vi "Main.vi"() -> ()   [LabVIEW 2026]
doc: "This template is for the Queued Message Handler design pattern.\n\nThe Event Handling Loop generates messages based on user interface actions.\n\nThe Message Handling Loop processes messages generated by the Event Handling Loop, or by other messages. The messages are string values, so new messages can be added easily to the Message Cases case structure in the Message Handling Loop. Each message cluster can also provide an optional value for Message Data, which is a variant that can be converted to whatever message-specific data is required."
uses:
  SubVIs/Controls/PCO_Config.ctl
  SubVIs/Controls/UI Data.ctl
  <instrlib>/PCO_SDK/File Group 0/vi.lib/Excelitas PCO GmbH/pco.labview/camera/Camera.lvclass
  <instrlib>/PCO_SDK/File Group 0/vi.lib/Excelitas PCO GmbH/pco.labview/camera/Controls/binning.ctl
  SubVIs/QMH/Message Queue/Enqueue Message (Single).vi
  SubVIs/QMH/Message Queue/Message Queue.lvlib
  SubVIs/QMH/User Event - Stop/User Event - Stop.lvlib
panel:
  out "Image 2":T1(plugin-control)
  in  "Stop live":bool
  out "rawImage":u16[][](array[numeric])
  out "Recording On":bool
  in  "FFT?":bool
  in  "Grab":bool
  in  "Live":bool
  in  "PCO_Config":T2={"Exposure time (s)"=0.1, "TriggerMode"=0, "ROI X0"=1, "ROI Y0"=1, "ROI X1"=2048, "ROI Y1"=2048, "Binning"=1} {"TriggerMode" items=["auto sequence", "software trigger", "external exposure start", "external exposure control"]}
  out "Image dimensions (px)":dbl[](array[numeric])=[2048.0, 2048.0]
  out "description":T3={"serial"=14401698, "type"=5632, "sub_type"=0, "interface_type"=8, "bit_resolution"=16, "min_exposure_time_s"=2.1e-05, "max_exposure_time_s"=5.0, "min_exposure_step_s"=1.2136e-05, "min_delay_time_s"=0.0, "max_delay_time_s"=5.0, "min_delay_step_s"=2.5e-08, "min_width"=64, "min_height"=16, "max_width"=2048, "max_height"=2048, "roi_step_horz"=32, "roi_step_vert"=8, "roi_symmetric_horz"=FALSE, "roi_symmetric_vert"=FALSE, "has_timestamp_mode"=TRUE, "has_timestamp_mode_ascii_only"=TRUE, "pixelrate_vec"=[44000000, 0, 0, 0], "has_acquire_mode"=TRUE, "has_ext_acquire_mode"=FALSE, "has_metadata_mode"=TRUE, "has_ram"=FALSE, "binning_horz_vec"=[1, 2, 4], "binning_vert_vec"=[1, 2, 4], "has_average_binning"=FALSE, "pixel_format_vec"=[1], "has_trigger_mode_extexpctrl"=TRUE} {"interface_type" items=["FireWire"=1, "GenICam"=3, "GigE"=5, "USB"=6, "CameraLinkME4"=7, "USB3"=8, "CLHS"=11, "All"=65535]}
  out "Current task":string="\"Exit\" button pressed"
  in  "Exit":bool
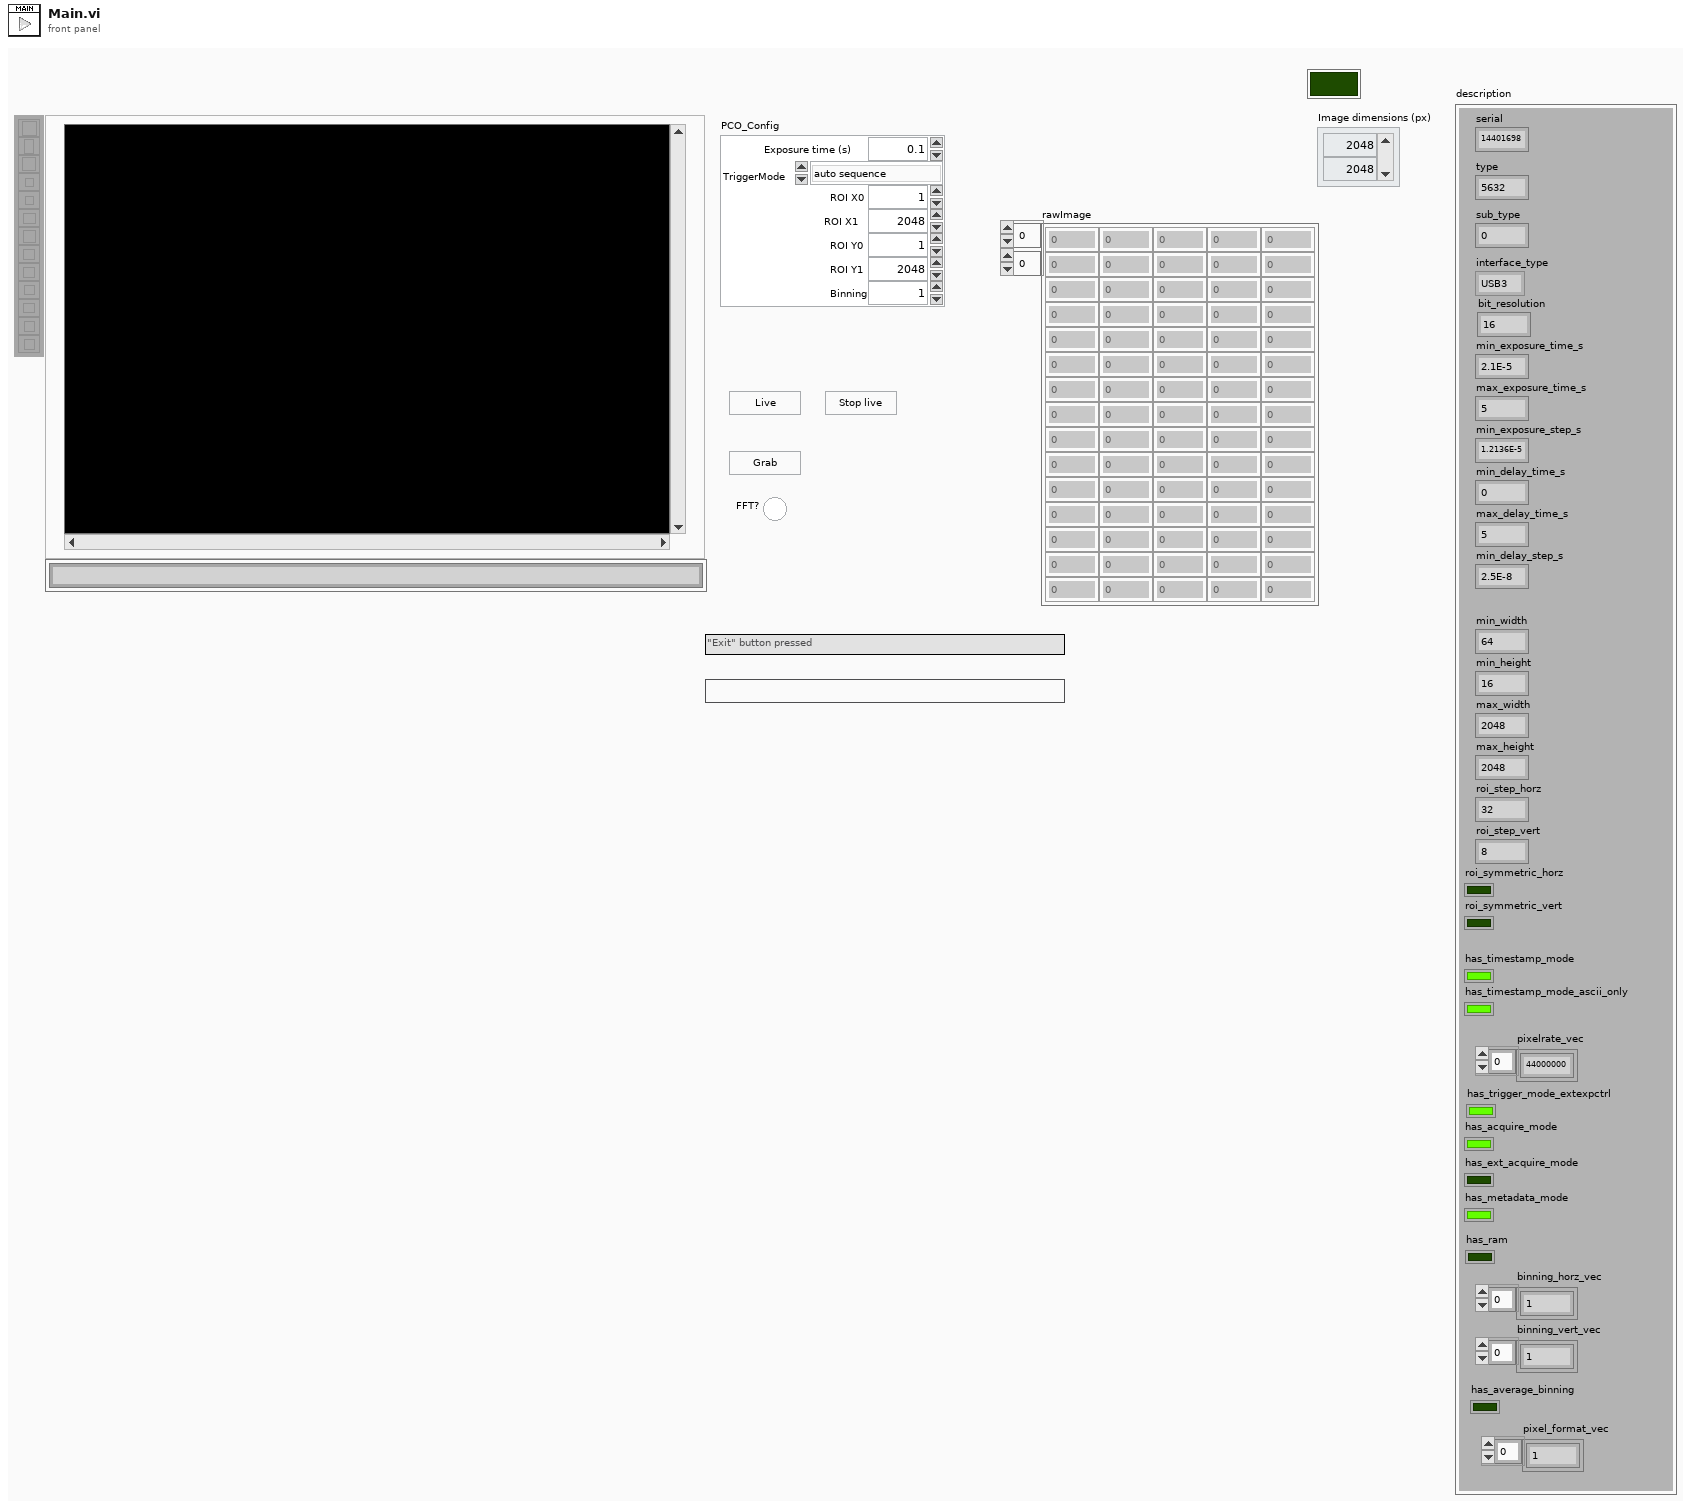
[diagram p1: front panel]
types:
  T1 = typedef "IMAQ Image.ctl" = refnum<image>
  T2 = typedef "PCO_Config.ctl" = cluster{"Exposure time (s)":dbl, "TriggerMode":u16, "ROI X0":u16, "ROI Y0":u16, "ROI X1":u16, "ROI Y1":u16, "Binning":u8}
  T3 = cluster{"serial":u32, "type":u16, "sub_type":u16, "interface_type":u16, "bit_resolution":u16, "min_exposure_time_s":dbl, "max_exposure_time_s":dbl, "min_exposure_step_s":dbl, "min_delay_time_s":dbl, "max_delay_time_s":dbl, "min_delay_step_s":dbl, "min_width":u64, "min_height":u64, "max_width":u64, "max_height":u64, "roi_step_horz":u64, "roi_step_vert":u64, "roi_symmetric_horz":bool, "roi_symmetric_vert":bool, "has_timestamp_mode":bool, "has_timestamp_mode_ascii_only":bool, "pixelrate_vec":u32[], "has_acquire_mode":bool, "has_ext_acquire_mode":bool, "has_metadata_mode":bool, "has_ram":bool, "binning_horz_vec":u16[], "binning_vert_vec":u16[], "has_average_binning":bool, "pixel_format_vec":u32[], "has_trigger_mode_extexpctrl":bool}
  T4 = typedef "UI Data.ctl" = cluster{"Data Display Ref":refnum<vi>, "Exit Button Ref":refnum<vi>, "Message":string}
  T5 = typedef "Message Queue.lvlib/All Message Queues.ctl" = cluster{"UI":refnum<queue>, "Camera loop":refnum<queue>, "Display loop":refnum<queue>}
  T6 = typedef "Camera.lvclass/binning.ctl" = cluster{"vert":u16, "horz":u16, "mode":u16}
  T7 = cluster{"exposure_time_s":dbl, "delay_time_s":dbl, "roi":cluster{"x0":u64, "y0":u64, "x1":u64, "y1":u64}, "timestamp_mode":u16, "pixelrate":u32, "trigger_mode":u16, "acquire_mode":u16, "metadata_mode":u16, "noisefilter_mode":u16, "pixel_format":u32, "binning":T6, "auto_exposure":cluster{"region":u16, "min_exposure_s":dbl, "max_exposure_s":dbl}}
  T8 = enum16{"sequence", "sequence non blocking", "ring buffer", "fifo", "sequence_dpcore", "sequence_non_blocking_dpcore", "ring_buffer_dpcore", "fifo_dpcore", "tif", "multitif", "pcoraw", "b16", "dicom", "multidicom", "camram_ring", "camram_segment"}
  T9 = enum16{"Undefined", "Mono8", "Mono16", "BGRA8", "RGBA8", "BGRA16", "RGBA16", "CompressedMono8"}
  T10 = typedef "Image Type" = u32
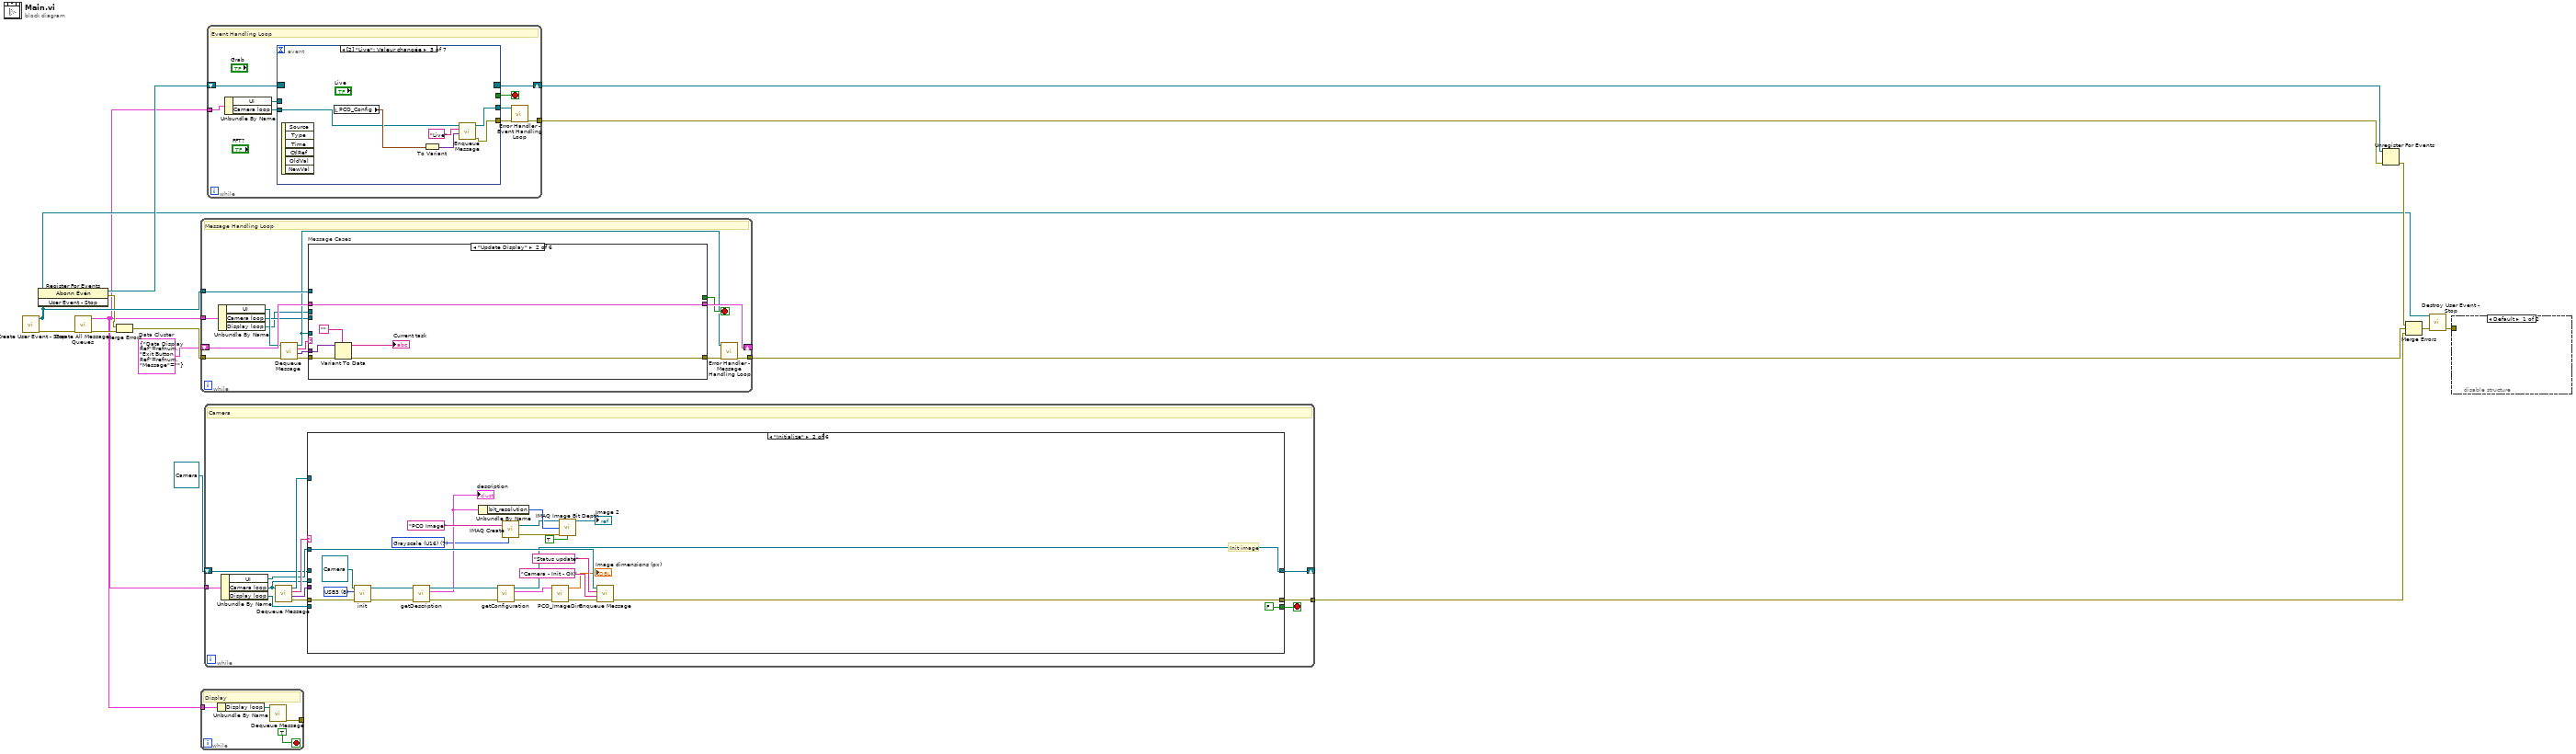
[diagram p0: block diagram]
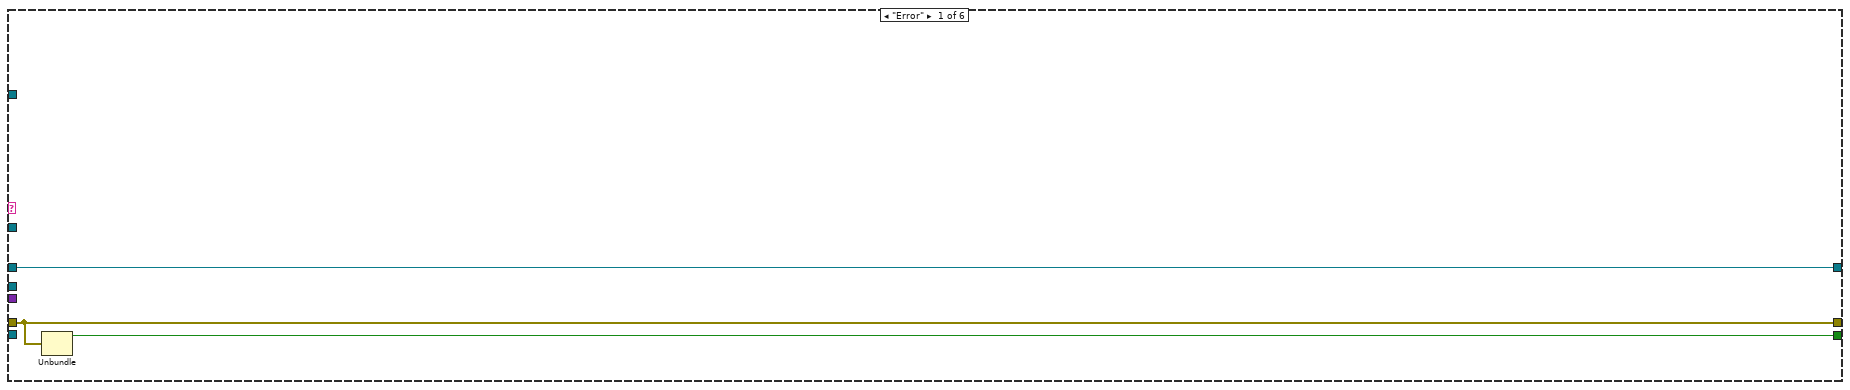
[diagram p2: hidden frame]
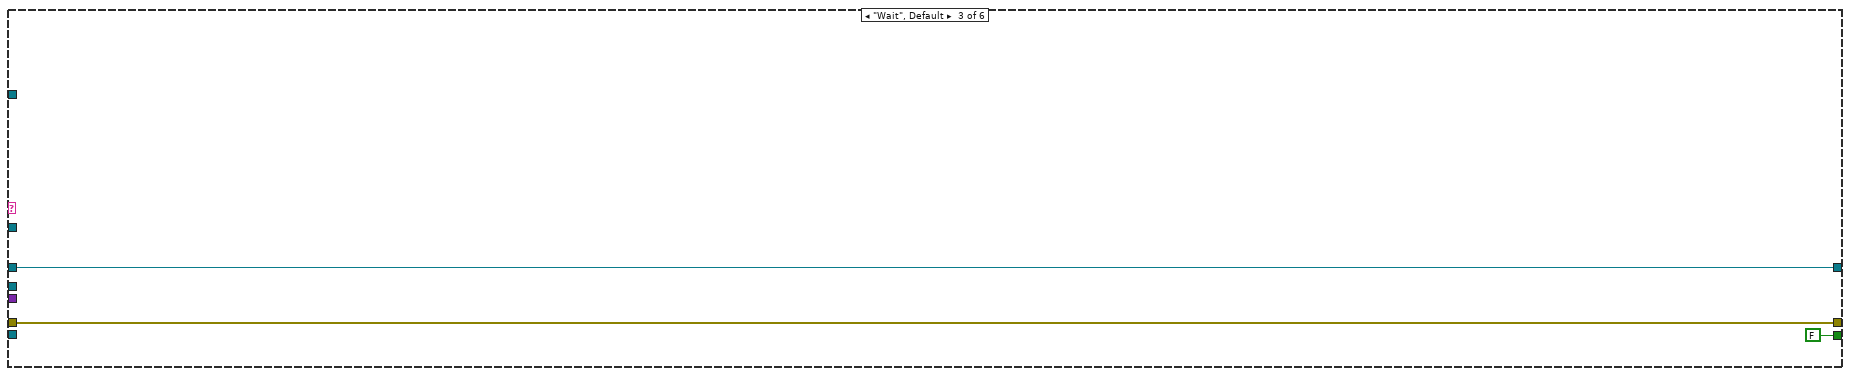
[diagram p3: hidden frame]
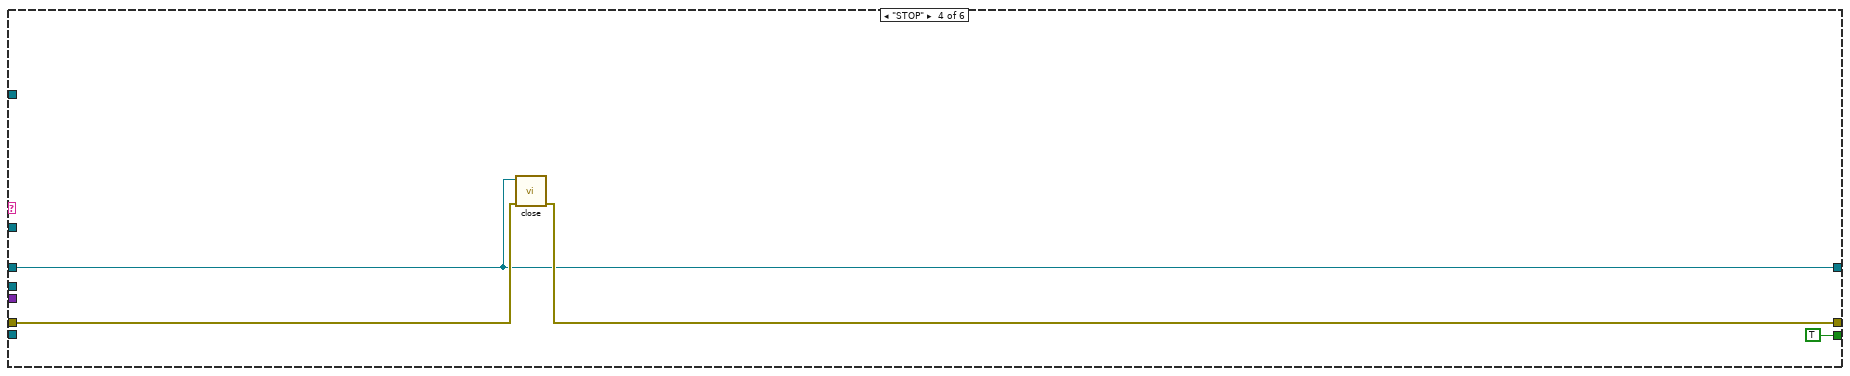
[diagram p4: hidden frame]
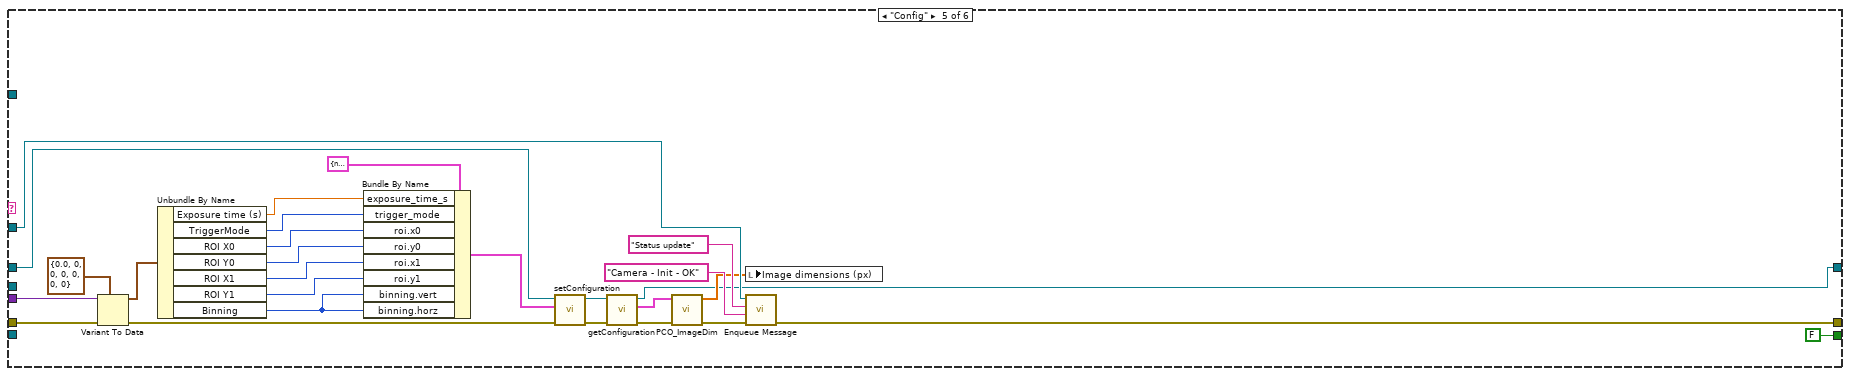
[diagram p5: hidden frame]
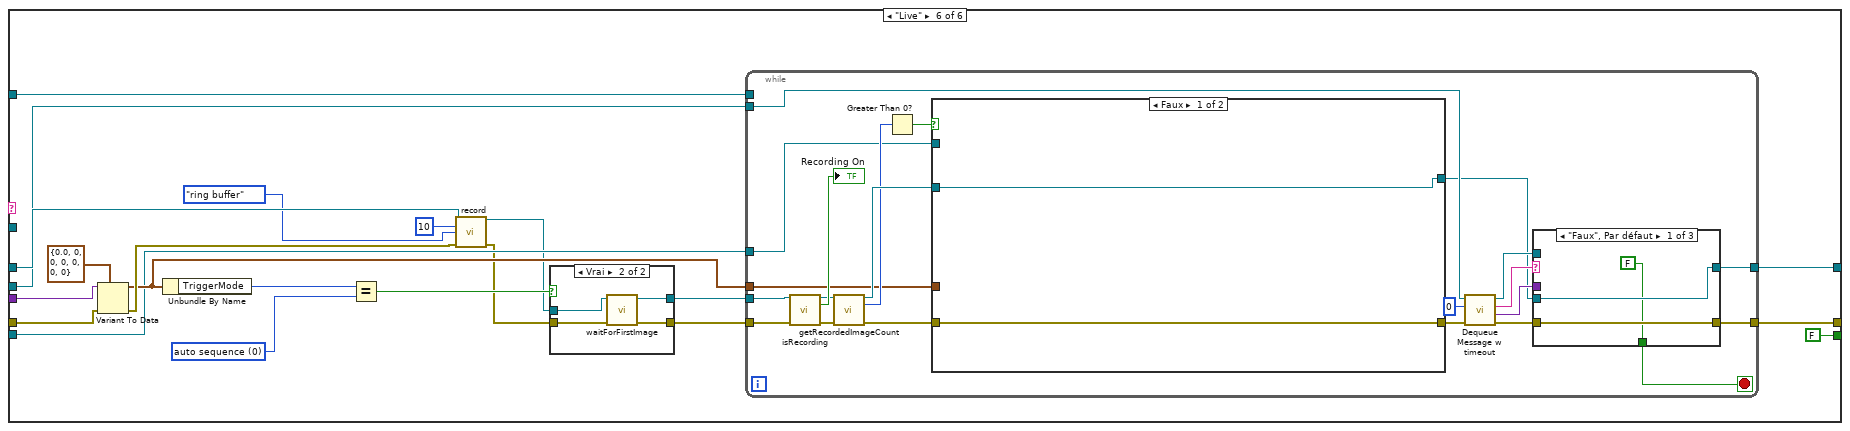
[diagram p6: hidden frame]
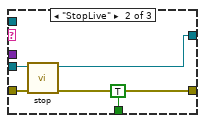
[diagram p7: hidden frame]
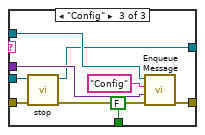
[diagram p8: hidden frame]
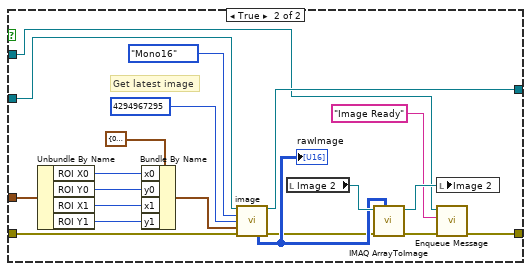
[diagram p9: hidden frame]
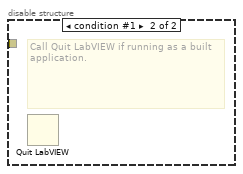
[diagram p11: hidden frame]
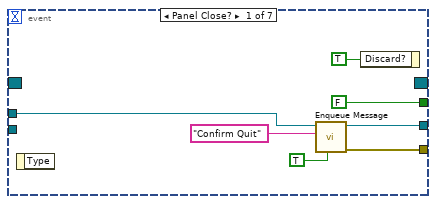
[diagram p12: hidden frame]
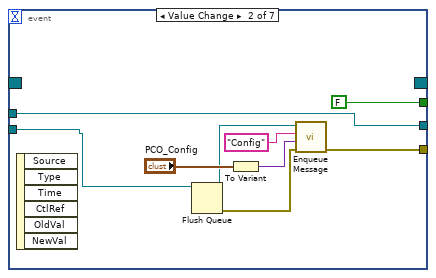
[diagram p13: hidden frame]
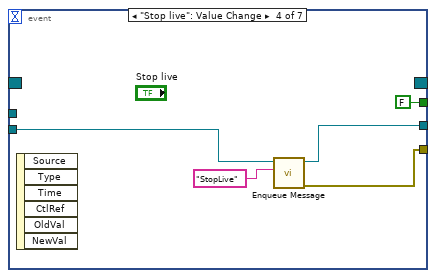
[diagram p14: hidden frame]
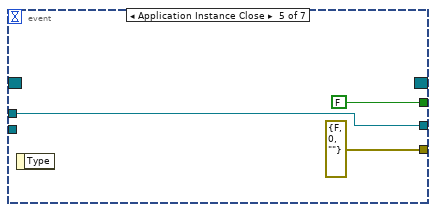
[diagram p15: hidden frame]
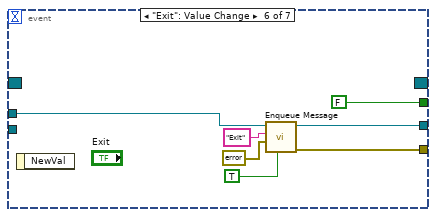
[diagram p16: hidden frame]
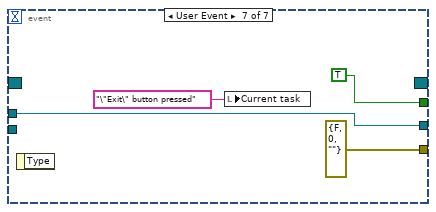
[diagram p17: hidden frame]
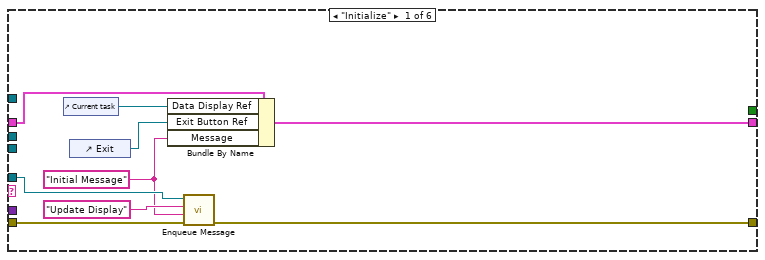
[diagram p18: hidden frame]
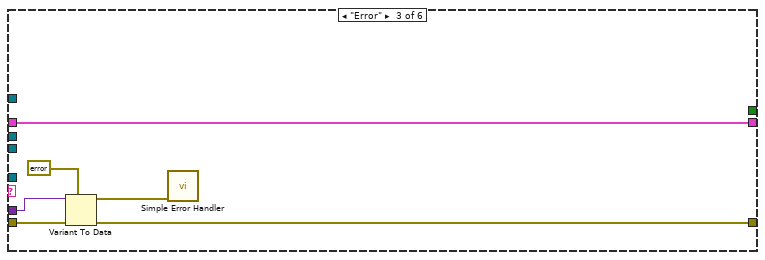
[diagram p19: hidden frame]
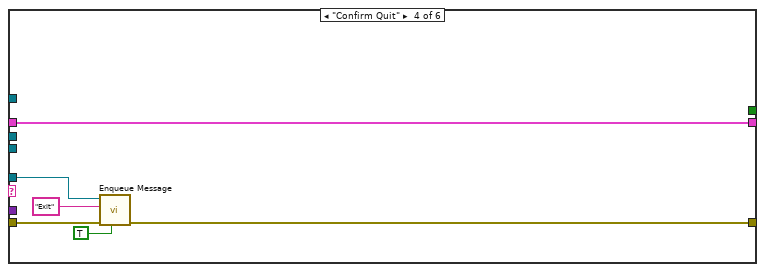
[diagram p20: hidden frame]
diagram:
  w4 = T4 {"Data Display Ref"=refnum, "Exit Button Ref"=refnum, "Message"=""}  # Data Cluster
  n1 = call "Create User Event - Stop.vi"() -> ("error out"=w14:errorcluster, "User Event - Stop"=w7:refnum<user-event>)  [unwired: 10 in]
  n2 = register-events(w7) -> (reference out=w8:refnum<event-registration>, error out=w5:errorcluster)  [unwired: 2 in]
  n3 = call "Create All Message Queues.vi"("error in (no error)"=w14) -> ("error out"=w16:errorcluster, "Message Queues out"=w2:T5)  [unwired: 9 in]
  n4 = Merge Errors(w5, w16) -> (w6:errorcluster)
  n5 = while {
    tunnel: [w18] -> _
    tunnel: w2 -> [w20]
    stop <- TRUE stop-if-true
    # "Display"
    n6 = Unbundle By Name(w20) -> ("Display loop"=w19:refnum<queue>)
    n7 = call "Dequeue Message.vi"("Message Queue"=w19) -> ("error out"=w18:errorcluster)  [unwired: 7 in, 3 out]
  }
  n8 = while {
    shift-right: [w34] -> _
    shift-left: w4 -> [w35]
    tunnel: w7 -> [w32]
    tunnel: w6 -> [w31]
    tunnel: [w26] -> w15
    tunnel: w2 -> [w24]
    stop <- w33 stop-if-true
    # "Message Handling Loop"
    n9 = Unbundle By Name(w24) -> ("UI"=w23:refnum<queue>, "Camera loop"=w22:refnum<queue>, "Display loop"=w21:refnum<queue>)
    n10 = call "Dequeue Message.vi"("error in (no error)"=w31, "Message Queue"=w23) -> ("error out"=w30:errorcluster, "Message Data"=w28:variant, "Message"=w29:string, "dup Message Queue"=w27:refnum<queue>)  [unwired: 6 in]
    n11 = case "Message Cases" shown="\"Update Display\"" w29 {
      tunnel: w27 -> [w38 _ _ w60 w74 _]
      tunnel: w30 -> [w43 w49 w56 w62 w75 w83]
      tunnel: [w44 w46 w51 w57 w70 w83] -> w25
      tunnel: w35 -> [w42 w50 w55 w61 w82 w84]
      tunnel: [w41 w50 w55 w61 w82 w84] -> w34
      tunnel: [_ _ _ _ TRUE _] -> w33
      tunnel: w28 -> [_ w48 w54 _ w78 _]
      tunnel: w32 -> [_ _ _ _ w80 _]
      tunnel: w22 -> [_ _ _ _ w73 _]
      tunnel: w21 -> [_ _ _ _ w63 _]
      frame "Initialize" {
        w36 = "Initial Message" ("Initial Message")
        n12 = control-ref of="Current task"() -> (w37:refnum<vi>)
        n13 = control-ref of="Exit"() -> (w40:refnum<vi>)
        n14 = Bundle By Name(cluster=w42, "Data Display Ref"=w37, "Exit Button Ref"=w40, "Message"=w36) -> (w41:T4)
        n15 = call-poly "Enqueue Message.vi"("error in (no error)"=w43, "Message Data"=w36, "Message"="Update Display", "Message Queue"=w38) -> ("error out"=w44:errorcluster)  [unwired: 6 in, 1 out]
      }
      frame "Update Display" {
        n16 = Variant To Data(error in=w49, type="", Variant=w48) -> (data=→"Current task":string, error out=w46:errorcluster)
      }
      frame "Error" {
        n17 = Variant To Data(error in=w56, type=errorcluster {"status"=FALSE, "code"=0, "source"=""} ("error constant"), Variant=w54) -> (data=w52:errorcluster, error out=w51:errorcluster)
        n18 = call <vilib>:"Simple Error Handler.vi"("error in (no error)"=w52) -> ()  [unwired: 4 in, 5 out]
      }
      frame "Confirm Quit" {
        n19 = call-poly "Enqueue Message.vi"("Priority Message? (F)"=TRUE, "error in (no error)"=w62, "Message"="Exit", "Message Queue"=w60) -> ("error out"=w57:errorcluster)  [unwired: 6 in, 1 out]
      }
      frame "Exit" {
        n20 = Variant To Data(error in=w75, type=errorcluster {"status"=FALSE, "code"=0, "source"=""} ("error constant"), Variant=w78) -> (error out=w71:errorcluster)  [unwired: 1 out]
        n21 = Release Queue(queue=w74, error in (no error)=w71) -> (error out=w69:errorcluster)  [unwired: 1 in, 2 out]
        n22 = call-poly "Enqueue Message.vi"("error in (no error)"=w69, "Message"="STOP", "Message Queue"=w73) -> ("error out"=w77:errorcluster, "dup Message Queue"=w76:refnum<queue>)  [unwired: 7 in]
        n23 = Release Queue(queue=w76, error in (no error)=w77) -> (error out=w65:errorcluster)  [unwired: 1 in, 2 out]
        n24 = call-poly "Enqueue Message.vi"("error in (no error)"=w65, "Message"="STOP", "Message Queue"=w63) -> ("error out"=w66:errorcluster, "dup Message Queue"=w67:refnum<queue>)  [unwired: 7 in]
        n25 = Release Queue(queue=w67, error in (no error)=w66) -> (error out=w64:errorcluster)  [unwired: 1 in, 2 out]
        n26 = call "Fire User Event - Stop.vi"("error in (no error)"=w64, "User Event - Stop"=w80) -> ("error out"=w70:errorcluster)  [unwired: 9 in]
      }
      frame Default {
      }
    }
    n27 = call "Error Handler - Message Handling Loop.vi"("error in (no error)"=w25, "Message Queue"=w27) -> ("dup error in"=w26:errorcluster)  [unwired: 8 in, 1 out]
  }
  n28 = while {
    tunnel: [w92] -> w3
    tunnel: w2 -> [w90]
    shift-right: [w88] -> _
    shift-left: refnum<class "Camera.lvclass"> refnum ("Camera out") -> [w87]
    stop <- w93 stop-if-true
    # "Camera"
    n29 = Unbundle By Name(w90) -> ("UI"=w89:refnum<queue>, "Camera loop"=w86:refnum<queue>, "Display loop"=w85:refnum<queue>)
    n30 = call "Dequeue Message.vi"("Message Queue"=w86) -> ("error out"=w96:errorcluster, "Message Data"=w94:variant, "Message"=w95:string, "dup Message Queue"=w91:refnum<queue>)  [unwired: 7 in]
    n31 = case shown="\"Initialize\"" w95 {
      tunnel: w96 -> [w99 w117 w127 w130 w157 w174]
      tunnel: w94 -> [_ _ _ _ w156 w170]
      tunnel: w89 -> [_ w124 _ _ w141 _]
      tunnel: [w98 FALSE ("status") FALSE ("status") TRUE FALSE ("status") FALSE ("status")] -> w93
      tunnel: [w99 w108 w127 w129 w140 w162] -> w92
      tunnel: w91 -> [_ _ _ _ _ w165]
      tunnel: [w97 w113 w126 w128 w132 w161] -> w88
      tunnel: w87 -> [w97 _ w126 w128 w151 w178]
      tunnel: w86 -> [_ _ _ _ _ w164]
      tunnel: w85 -> [_ _ _ _ _ w163]
      frame "Error" {
        n32 = Unbundle(w99) -> ("status"=w98:bool)  [unwired: 2 out]
      }
      frame "Initialize" {
        w103 = T10 7 items=["Grayscale (U8)", "Grayscale (I16)", "Grayscale (SGL)", "Complex (CSG)", "RGB (U32)", "HSL (U32)", "RGB (U64)", "Grayscale (U16)"] ("Image Type")
        w116 = u16 8 items=["FireWire"=1, "GenICam"=3, "GigE"=5, "USB"=6, "CameraLinkME4"=7, "USB3"=8, "CLHS"=11, "All"=65535] ("interface")
        # "Init image"
        n33 = call-dynamic "init.vi"("Camera in"=refnum<class "Camera.lvclass"> refnum, "interface"=w116, "error in (no error)"=w117) -> ("Camera out"=w120:refnum<class "Camera.lvclass">, "error out"=w119:errorcluster)  [unwired: 6 in]
        n34 = call-dynamic "getDescription.vi"("error in (no error)"=w119, "Camera in"=w120) -> ("error out"=w115:errorcluster, "description"=w105:T3, "Camera out"=w114:refnum<class "Camera.lvclass">)  [unwired: 7 in]
        "description" <- w105
        n35 = Unbundle By Name(w105) -> ("bit_resolution"=w104:u16)
        n36 = call-dynamic "getConfiguration.vi"("error in (no error)"=w115, "Camera in"=w114) -> ("error out"=w111:errorcluster, "configuration"=w112:T7, "Camera out"=w113:refnum<class "Camera.lvclass">)  [unwired: 7 in]
        n37 = call "IMAQ Create"("Image Name"="PCO Image", "Image Type"=w103) -> ("New Image"=w101:T1, "error out"=w100:errorcluster)  [unwired: 3 in]
        n38 = call "PCO_ImageDim.vi"("error in"=w111, "configuration"=w112) -> ("error out"=w110:errorcluster, "Dimensions"=→"Image dimensions (px)":dbl[])  [unwired: 8 in]
        n39 = call "IMAQ Image Bit Depth"("Image"=w101, "Bit Depth (0)"=w104, "error in (no error)"=w100, "Get/Set Bit Depth? (Set)"=TRUE) -> ("Image Out"=→"Image 2":T1)  [unwired: 9 in, 2 out]
        n40 = call-poly "Enqueue Message.vi"("error in (no error)"=w110, "Message Data"="Camera - Init - OK", "Message"="Status update", "Message Queue"=w124) -> ("error out"=w108:errorcluster)  [unwired: 6 in, 1 out]
      }
      frame "Wait", Default {
      }
      frame "STOP" {
        n41 = call-dynamic "close.vi"("error in (no error)"=w130, "Camera in"=w128) -> ("error out"=w129:errorcluster)  [unwired: 9 in]
      }
      frame "Config" {
        n42 = Variant To Data(error in=w157, type=T2 {"Exposure time (s)"=0.0, "TriggerMode"=0, "ROI X0"=0, "ROI Y0"=0, "ROI X1"=0, "ROI Y1"=0, "Binning"=0} ("PCO_Config"), Variant=w156) -> (data=w153:T2, error out=w152:errorcluster)
        n43 = Unbundle By Name(w153) -> ("Exposure time (s)"=w149:dbl, "TriggerMode"=w148:u16, "ROI X0"=w143:u16, "ROI Y0"=w144:u16, "ROI X1"=w145:u16, "ROI Y1"=w146:u16, "Binning"=w147:u8)
        n44 = Bundle By Name(cluster=T7 {"exposure_time_s"=nan, "delay_time_s"=nan, "roi"={"x0"=18446744073709551615, "y0"=18446744073709551615, "x1"=18446744073709551615, "y1"=18446744073709551615}, "timestamp_mode"=65535, "pixelrate"=4294967295, "trigger_mode"=65535, "acquire_mode"=65535, "metadata_mode"=65535, "noisefilter_mode"=65535, "pixel_format"=4294967295, "binning"={"vert"=65535, "horz"=65535, "mode"=0}, "auto_exposure"={"region"=0, "min_exposure_s"=0.001, "max_exposure_s"=0.1}} ("configuration"), "exposure_time_s"=w149, "trigger_mode"=w148, "roi.x0"=w143, "roi.y0"=w144, "roi.x1"=w145, "roi.y1"=w146, "binning.vert"=w147, "binning.horz"=w147) -> (w150:T7)
        n45 = call-dynamic "setConfiguration.vi"("error in (no error)"=w152, "configuration"=w150, "Camera in"=w151) -> ("error out"=w134:errorcluster, "Camera out"=w135:refnum<class "Camera.lvclass">)  [unwired: 7 in]
        n46 = call-dynamic "getConfiguration.vi"("error in (no error)"=w134, "Camera in"=w135) -> ("error out"=w138:errorcluster, "configuration"=w137:T7, "Camera out"=w132:refnum<class "Camera.lvclass">)  [unwired: 7 in]
        n47 = call "PCO_ImageDim.vi"("error in"=w138, "configuration"=w137) -> ("error out"=w133:errorcluster, "Dimensions"=w136:dbl[])  [unwired: 8 in]
        n48 = local write "Image dimensions (px)"(w136) -> ()
        n49 = call-poly "Enqueue Message.vi"("error in (no error)"=w133, "Message Data"="Camera - Init - OK", "Message"="Status update", "Message Queue"=w141) -> ("error out"=w140:errorcluster)  [unwired: 6 in, 1 out]
      }
      frame "Live" {
        w172 = u16 0 items=["auto sequence", "software trigger", "external exposure start", "external exposure control"] ("TriggerMode")
        n50 = Variant To Data(error in=w174, type=T2 {"Exposure time (s)"=0.0, "TriggerMode"=0, "ROI X0"=0, "ROI Y0"=0, "ROI X1"=0, "ROI Y1"=0, "Binning"=0} ("PCO_Config"), Variant=w170) -> (data=w166:T2, error out=w173:errorcluster)
        n51 = Unbundle By Name(w166) -> ("TriggerMode"=w171:u16)
        n52 = Equal?(x=w171, y=w172) -> (x = y?=w169:bool)
        n53 = call-dynamic "record.vi"("Camera in"=w178, "num_images"=u32 10 ("dwImgCount"), "record_mode"=T8."ring buffer", "error in (no error)"=w173) -> ("Camera out"=w159:refnum<class "Camera.lvclass">, "error out"=w160:errorcluster)  [unwired: 10 in]
        n54 = case shown="Vrai" w169 {
          tunnel: w160 -> [w241 w246]
          tunnel: w159 -> [w242 w245]
          tunnel: [w242 w244] -> w167
          tunnel: [w241 w243] -> w168
          frame False {
          }
          frame True {
            n55 = call-dynamic "waitForFirstImage.vi"("error in (no error)"=w246, "Camera in"=w245) -> ("error out"=w243:errorcluster, "Camera out"=w244:refnum<class "Camera.lvclass">)  [unwired: 8 in]
          }
        }
        n56 = while {
          tunnel: w168 -> [w194]
          tunnel: w167 -> [w193]
          tunnel: w166 -> [w192]
          tunnel: w165 -> [_]
          tunnel: w164 -> [w190]
          tunnel: w163 -> [w188]
          tunnel: [w183] -> w162
          tunnel: [w182] -> w161
          stop <- w181 stop-if-true
          n57 = call-dynamic "isRecording.vi"("Camera in"=w193, "error in (no error)"=w194) -> ("Camera out"=w200:refnum<class "Camera.lvclass">, "recording"=→"Recording On":bool, "error out"=w199:errorcluster)  [unwired: 11 in]
          n58 = call-dynamic "getRecordedImageCount.vi"("Camera in"=w200, "error in (no error)"=w199) -> ("Camera out"=w197:refnum<class "Camera.lvclass">, "recorded_image_count"=w195:u32, "error out"=w198:errorcluster)  [unwired: 11 in]
          n59 = Greater Than 0?(x=w195) -> (x > 0?=w196:bool)
          n60 = case shown="Faux" w196 {
            tunnel: [w219 w223] -> w191
            tunnel: w198 -> [w219 w237]
            tunnel: w197 -> [w220 w233]
            tunnel: [w220 w232] -> w184
            tunnel: w192 -> [_ w231]
            tunnel: w188 -> [_ w225]
            frame False {
            }
            frame True {
              # "Get latest image"
              n61 = Unbundle By Name(w231) -> ("ROI X0"=w230:u16, "ROI Y0"=w229:u16, "ROI X1"=w228:u16, "ROI Y1"=w227:u16)
              n62 = Bundle By Name(cluster=cluster{"x0":u64, "y0":u64, "x1":u64, "y1":u64} {"x0"=0, "y0"=0, "x1"=0, "y1"=0} ("roi"), "x0"=w230, "y0"=w229, "x1"=w228, "y1"=w227) -> (w238:cluster{"x0":u64, "y0":u64, "x1":u64, "y1":u64})
              n63 = call-dynamic "image.vi"("Camera in"=w233, "data_format"=T9."Mono16", "image_index"=u32 4294967295 ("dwImgIdx"), "roi"=w238, "error in (no error)"=w237) -> ("Camera out"=w232:refnum<class "Camera.lvclass">, "raw_image (U16)"=w234:u16[][], "error out"=w222:errorcluster)  [unwired: 2 in, 6 out]
              "rawImage" <- w234
              n64 = local read "Image 2"() -> (w235:T1)
              n65 = call "IMAQ ArrayToImage"("Image Pixels (U16)"=w234, "error in (no error)"=w222, "Image"=w235) -> ("error out"=w221:errorcluster, "Image Out"=w236:T1)  [unwired: 7 in]
              n66 = local write "Image 2"(w236) -> ()
              n67 = call-poly "Enqueue Message.vi"("error in (no error)"=w221, "Message"="Image Ready", "Message Queue"=w225) -> ("error out"=w223:errorcluster)  [unwired: 7 in, 1 out]
            }
          }
          n68 = call "Dequeue Message w timeout.vi"("entrée d'erreur (pas d'erreur)"=w191, "timeout en ms (-1)"=0, "Message Queue"=w190) -> ("sortie d'erreur"=w186:errorcluster, "Message Data"=w185:variant, "Message"=w189:string, "Message Queue"=w187:refnum<queue>)  [unwired: 5 in]
          n69 = case shown="\"Faux\", Par défaut" w189 {
            tunnel: w187 -> [_ _ w218]
            tunnel: w186 -> [w203 w208 w213]
            tunnel: w185 -> [_ _ w216]
            tunnel: w184 -> [w204 w209 w214]
            tunnel: [w203 w207 w211] -> w183
            tunnel: [w204 w206 w215] -> w182
            tunnel: [FALSE TRUE FALSE] -> w181
            frame "Faux", Default {
            }
            frame "StopLive" {
              n70 = call-dynamic "stop.vi"("error in (no error)"=w208, "Camera in"=w209) -> ("error out"=w207:errorcluster, "Camera out"=w206:refnum<class "Camera.lvclass">)  [unwired: 8 in]
            }
            frame "Config" {
              n71 = call-dynamic "stop.vi"("error in (no error)"=w213, "Camera in"=w214) -> ("error out"=w212:errorcluster, "Camera out"=w215:refnum<class "Camera.lvclass">)  [unwired: 8 in]
              n72 = call-poly "Enqueue Message.vi"("error in (no error)"=w212, "Message Data"=w216, "Message"="Config", "Message Queue"=w218) -> ("error out"=w211:errorcluster)  [unwired: 6 in, 1 out]
            }
          }
        }
      }
    }
  }
  n73 = while {
    shift-right: [w254] -> w11
    shift-left: w8 -> [w255]
    tunnel: [w250] -> w9
    tunnel: w2 -> [w247]
    stop <- w252 stop-if-true
    # "Event Handling Loop"
    n74 = Unbundle By Name(w247) -> ("UI"=w249:refnum<queue>, "Camera loop"=w248:refnum<queue>)
    n75 = event shown="[2] \"Live\": Valeur changée" {
      selector: w255 -> [_ _ _ _ _ _ _]
      dyn-events: [_ _ _ _ _ _ _] -> w254
      timeout: _ -> [_ _ _ _ _ _ _]
      tunnel: [FALSE ("Discard?") FALSE ("Discard?") _ FALSE ("Discard?") FALSE ("Discard?") FALSE ("Discard?") TRUE ("Discard?")] -> w252
      tunnel: w249 -> [w261 w271 _ _ w285 w292 w296]
      tunnel: [w260 w267 w274 w280 errorcluster {"status"=FALSE, "code"=0, "source"=""} ("error out") w286 errorcluster {"status"=FALSE, "code"=0, "source"=""} ("error out")] -> w253
      tunnel: [w259 w271 w273 w279 w285 w291 w296] -> w251
      tunnel: w248 -> [_ w265 w272 w281 _ _ _]
      event Panel Close? {
        n76 = event-data() -> ()  [unwired: 1 in, 1 out]
        n77 = call-poly "Enqueue Message.vi"("Priority Message? (F)"=TRUE, "Message"="Confirm Quit", "Message Queue"=w261) -> ("error out"=w260:errorcluster, "dup Message Queue"=w259:refnum<queue>)  [unwired: 7 in]
        n78 = event-data("Discard?"=TRUE) -> ()  [unwired: 1 in, 1 out]
      }
      event Value Change {
        n79 = event-data() -> ()  [unwired: 1 in, 6 out]
        n80 = Flush Queue(queue=w265) -> (queue out=w263:refnum<queue>, error out=w264:errorcluster)  [unwired: 1 in, 1 out]
        n81 = To Variant(anything="PCO_Config") -> (Variant=w268:variant)
        n82 = call-poly "Enqueue Message.vi"("error in (no error)"=w264, "Message Data"=w268, "Message"="Config", "Message Queue"=w263) -> ("error out"=w267:errorcluster)  [unwired: 6 in, 1 out]
      }
      event "Live": Value Change {
        n83 = event-data() -> ()  [unwired: 1 in, 6 out]
        n84 = local read "PCO_Config"() -> (w277:T2)
        n85 = To Variant(anything=w277) -> (Variant=w276:variant)
        n86 = call-poly "Enqueue Message.vi"("Message Data"=w276, "Message"="Live", "Message Queue"=w272) -> ("error out"=w274:errorcluster, "dup Message Queue"=w273:refnum<queue>)  [unwired: 7 in]
      }
      event "Stop live": Value Change {
        n87 = event-data() -> ()  [unwired: 1 in, 6 out]
        n88 = call-poly "Enqueue Message.vi"("Message"="StopLive", "Message Queue"=w281) -> ("error out"=w280:errorcluster, "dup Message Queue"=w279:refnum<queue>)  [unwired: 8 in]
      }
      event Application Instance Close {
        n89 = event-data() -> ()  [unwired: 1 in, 1 out]
      }
      event "Exit": Value Change {
        n90 = event-data() -> ()  [unwired: 1 in, 1 out]
        n91 = call-poly "Enqueue Message.vi"("Priority Message? (F)"=TRUE, "Message Data"=errorcluster {"status"=FALSE, "code"=0, "source"=""} ("error constant"), "Message"="Exit", "Message Queue"=w292) -> ("error out"=w286:errorcluster, "dup Message Queue"=w291:refnum<queue>)  [unwired: 6 in]
      }
      event User Event {
        n92 = event-data() -> ()  [unwired: 1 in, 1 out]
        n93 = local write "Current task"("\"Exit\" button pressed" ("VI Stopped")) -> ()
      }
    }
    n94 = call "Error Handler - Event Handling Loop.vi"("error in (no error)"=w253, "Message Queue"=w251) -> ("dup error in"=w250:errorcluster)  [unwired: 8 in, 1 out]
  }
  n95 = Unregister For Events(event registration refnum=w11, error in=w9) -> (error out=w12:errorcluster)
  n96 = Merge Errors(w12, w15, w3) -> (w13:errorcluster)
  n97 = call "Destroy User Event - Stop.vi"("error in (no error)"=w13, "User Event - Stop"=w7) -> ("error out"=w10:errorcluster)  [unwired: 9 in]
  n98 = disable-structure shown="Default" {
    disable-tunnel: w10 -> [_ _]
    frame condition #0 (active) {
    }
    frame condition #1 {
      # "Call Quit LabVIEW if running as a built application."
      n99 = Quit LabVIEW() -> ()  [unwired: 1 in]
    }
  }
